vi "Lab Panel V5.27.vi"() -> ()   [LabVIEW 2013] (continued)
                            n3235 = Multiply(x=w5893, y=w5892) -> (x*y=w5891:dbl)
                            n3236 = Multiply(x=w5893, y=w5895) -> (x*y=w5894:dbl)
                          }
                        }
                        n3237 = local read "SIG LAB02-2"() -> (w5885:T2)
                        n3238 = local read "SIG LAB02-1"() -> (w5887:T2)
                        n3239 = Bundle By Name(cluster=w5887, "Tmp Live"=w5867, "Tmp Neut"=w5866) -> (w5886:T2)
                        n3240 = Bundle By Name(cluster=w5885, "Tmp Live"=w5863, "Tmp Neut"=w5862) -> (w5884:T2)
                        n3241 = local write "SIG LAB02-1"(w5886) -> ()
                        n3242 = local write "SIG LAB02-2"(w5884) -> ()
                      }
                      frame #3 {
                        n3243 = case shown="False" w5917 {
                          tunnel: [w5948 w5949] -> w5933
                          tunnel: w5916 -> [_ w5949]
                          frame False {
                            n3244 = local read "CAL LAB03"() -> (w5948:T14)
                          }
                          frame True {
                          }
                        }
                        n3245 = local read "TEMP LA03"() -> (w5923:T9)
                        n3246 = local read "LAB03 TEMP"() -> (w5924:T12)
                        n3247 = call "sub vi - temperature delay v4.vi"("2-run"=w5905, "1-run"=w5906, "temp values IN"=w5923, "temp signals"=w5924) -> ("T2-N"=w5918:dbl, "T2-L"=w5919:dbl, "T1-N"=w5920:dbl, "T1-L"=w5921:dbl, "temp values OUT"=w5922:T44)  [unwired: 3 in]
                        n3248 = Unbundle By Name(w5933) -> ("1 (TL) cal"=w5928:dbl, "1 (TN) cal"=w5927:dbl, "2 (TL) cal"=w5926:dbl, "2 (TN) cal"=w5925:dbl)  [unwired: 6 out]
                        n3249 = local write "TEMP LA03"(w5922) -> ()
                        n3250 = Multiply(x=w5921, y=w5928) -> (x*y=w5914:dbl)
                        n3251 = Multiply(x=w5920, y=w5927) -> (x*y=w5913:dbl)
                        n3252 = Multiply(x=w5919, y=w5926) -> (x*y=w5910:dbl)
                        n3253 = Multiply(x=w5918, y=w5925) -> (x*y=w5909:dbl)
                        n3254 = case shown="True" w5905 {
                          tunnel: w5910 -> [w5935 w5940]
                          tunnel: w5915 -> [_ w5938]
                          tunnel: [w5935 w5939] -> w5908
                          tunnel: w5909 -> [w5934 w5937]
                          tunnel: [w5934 w5936] -> w5907
                          frame False {
                          }
                          frame True {
                            n3255 = Multiply(x=w5938, y=w5937) -> (x*y=w5936:dbl)
                            n3256 = Multiply(x=w5938, y=w5940) -> (x*y=w5939:dbl)
                          }
                        }
                        n3257 = case shown="True" w5906 {
                          tunnel: w5914 -> [w5942 w5947]
                          tunnel: w5915 -> [_ w5945]
                          tunnel: [w5942 w5946] -> w5912
                          tunnel: w5913 -> [w5941 w5944]
                          tunnel: [w5941 w5943] -> w5911
                          frame False {
                          }
                          frame True {
                            n3258 = Multiply(x=w5945, y=w5944) -> (x*y=w5943:dbl)
                            n3259 = Multiply(x=w5945, y=w5947) -> (x*y=w5946:dbl)
                          }
                        }
                        n3260 = local read "SIG LAB03-2"() -> (w5930:T2)
                        n3261 = local read "SIG LAB03-1"() -> (w5932:T2)
                        n3262 = Bundle By Name(cluster=w5932, "Tmp Live"=w5912, "Tmp Neut"=w5911) -> (w5931:T2)
                        n3263 = Bundle By Name(cluster=w5930, "Tmp Live"=w5908, "Tmp Neut"=w5907) -> (w5929:T2)
                        n3264 = local write "SIG LAB03-1"(w5931) -> ()
                        n3265 = local write "SIG LAB03-2"(w5929) -> ()
                      }
                      frame #4 {
                        n3266 = case shown="False" w5962 {
                          tunnel: [w5993 w5994] -> w5978
                          tunnel: w5961 -> [_ w5994]
                          frame False {
                            n3267 = local read "CAL LAB04"() -> (w5993:T14)
                          }
                          frame True {
                          }
                        }
                        n3268 = local read "LAB04 TEMP"() -> (w5968:T12)
                        n3269 = local read "TEMP LA04"() -> (w5969:T9)
                        n3270 = call "sub vi - temperature delay v4.vi"("2-run"=w5950, "1-run"=w5951, "temp values IN"=w5969, "temp signals"=w5968) -> ("T2-N"=w5963:dbl, "T2-L"=w5964:dbl, "T1-N"=w5965:dbl, "T1-L"=w5966:dbl, "temp values OUT"=w5967:T44)  [unwired: 3 in]
                        n3271 = Unbundle By Name(w5978) -> ("1 (TL) cal"=w5973:dbl, "1 (TN) cal"=w5972:dbl, "2 (TL) cal"=w5971:dbl, "2 (TN) cal"=w5970:dbl)  [unwired: 6 out]
                        n3272 = local write "TEMP LA04"(w5967) -> ()
                        n3273 = Multiply(x=w5966, y=w5973) -> (x*y=w5959:dbl)
                        n3274 = Multiply(x=w5965, y=w5972) -> (x*y=w5958:dbl)
                        n3275 = Multiply(x=w5964, y=w5971) -> (x*y=w5955:dbl)
                        n3276 = Multiply(x=w5963, y=w5970) -> (x*y=w5954:dbl)
                        n3277 = case shown="True" w5950 {
                          tunnel: w5955 -> [w5980 w5985]
                          tunnel: w5960 -> [_ w5983]
                          tunnel: [w5980 w5984] -> w5953
                          tunnel: w5954 -> [w5979 w5982]
                          tunnel: [w5979 w5981] -> w5952
                          frame False {
                          }
                          frame True {
                            n3278 = Multiply(x=w5983, y=w5982) -> (x*y=w5981:dbl)
                            n3279 = Multiply(x=w5983, y=w5985) -> (x*y=w5984:dbl)
                          }
                        }
                        n3280 = case shown="True" w5951 {
                          tunnel: w5959 -> [w5987 w5992]
                          tunnel: w5960 -> [_ w5990]
                          tunnel: [w5987 w5991] -> w5957
                          tunnel: w5958 -> [w5986 w5989]
                          tunnel: [w5986 w5988] -> w5956
                          frame False {
                          }
                          frame True {
                            n3281 = Multiply(x=w5990, y=w5989) -> (x*y=w5988:dbl)
                            n3282 = Multiply(x=w5990, y=w5992) -> (x*y=w5991:dbl)
                          }
                        }
                        n3283 = local read "SIG LAB04-2"() -> (w5975:T2)
                        n3284 = local read "SIG LAB04-1"() -> (w5977:T2)
                        n3285 = Bundle By Name(cluster=w5977, "Tmp Live"=w5957, "Tmp Neut"=w5956) -> (w5976:T2)
                        n3286 = Bundle By Name(cluster=w5975, "Tmp Live"=w5953, "Tmp Neut"=w5952) -> (w5974:T2)
                        n3287 = local write "SIG LAB04-1"(w5976) -> ()
                        n3288 = local write "SIG LAB04-2"(w5974) -> ()
                      }
                      frame #5 {
                        n3289 = case shown="False" w6007 {
                          tunnel: [w6038 w6039] -> w6023
                          tunnel: w6006 -> [_ w6039]
                          frame False {
                            n3290 = local read "CAL LAB05"() -> (w6038:T14)
                          }
                          frame True {
                          }
                        }
                        n3291 = local read "LAB05 TEMP"() -> (w6013:T12)
                        n3292 = local read "TEMP LA05"() -> (w6014:T9)
                        n3293 = call "sub vi - temperature delay v4.vi"("2-run"=w5995, "1-run"=w5996, "temp values IN"=w6014, "temp signals"=w6013) -> ("T2-N"=w6009:dbl, "T2-L"=w6010:dbl, "T1-N"=w6011:dbl, "T1-L"=w6012:dbl, "temp values OUT"=w6008:T44)  [unwired: 3 in]
                        n3294 = local write "TEMP LA05"(w6008) -> ()
                        n3295 = Unbundle By Name(w6023) -> ("1 (TL) cal"=w6015:dbl, "1 (TN) cal"=w6018:dbl, "2 (TL) cal"=w6017:dbl, "2 (TN) cal"=w6016:dbl)  [unwired: 6 out]
                        n3296 = Multiply(x=w6012, y=w6015) -> (x*y=w6004:dbl)
                        n3297 = Multiply(x=w6011, y=w6018) -> (x*y=w6003:dbl)
                        n3298 = Multiply(x=w6010, y=w6017) -> (x*y=w6000:dbl)
                        n3299 = Multiply(x=w6009, y=w6016) -> (x*y=w5999:dbl)
                        n3300 = case shown="True" w5995 {
                          tunnel: w6000 -> [w6025 w6030]
                          tunnel: w6005 -> [_ w6028]
                          tunnel: [w6025 w6029] -> w5998
                          tunnel: w5999 -> [w6024 w6027]
                          tunnel: [w6024 w6026] -> w5997
                          frame False {
                          }
                          frame True {
                            n3301 = Multiply(x=w6028, y=w6027) -> (x*y=w6026:dbl)
                            n3302 = Multiply(x=w6028, y=w6030) -> (x*y=w6029:dbl)
                          }
                        }
                        n3303 = case shown="True" w5996 {
                          tunnel: w6004 -> [w6032 w6037]
                          tunnel: w6005 -> [_ w6035]
                          tunnel: [w6032 w6036] -> w6002
                          tunnel: w6003 -> [w6031 w6034]
                          tunnel: [w6031 w6033] -> w6001
                          frame False {
                          }
                          frame True {
                            n3304 = Multiply(x=w6035, y=w6034) -> (x*y=w6033:dbl)
                            n3305 = Multiply(x=w6035, y=w6037) -> (x*y=w6036:dbl)
                          }
                        }
                        n3306 = local read "SIG LAB05-1"() -> (w6022:T2)
                        n3307 = Bundle By Name(cluster=w6022, "Tmp Live"=w6002, "Tmp Neut"=w6001) -> (w6021:T2)
                        n3308 = local read "SIG LAB05-2"() -> (w6020:T2)
                        n3309 = Bundle By Name(cluster=w6020, "Tmp Live"=w5998, "Tmp Neut"=w5997) -> (w6019:T2)
                        n3310 = local write "SIG LAB05-1"(w6021) -> ()
                        n3311 = local write "SIG LAB05-2"(w6019) -> ()
                      }
                      frame #6 {
                        w6140 = 150.0
                        # "check for thermocouple error, output >150 deg??"
                        n3312 = local read "SIG LAB01-2"() -> (w6149:T2)
                        n3313 = local read "SIG LAB04-1"() -> (w6143:T2)
                        n3314 = local read "SIG LAB04-2"() -> (w6144:T2)
                        n3315 = local read "SIG LAB01-1"() -> (w6150:T2)
                        n3316 = Unbundle(w6144) -> ("Tmp Live"=w6054:dbl, "Tmp Neut"=w6053:dbl)  [unwired: 3 out]
                        n3317 = Unbundle(w6149) -> ("Tmp Live"=w6075:dbl, "Tmp Neut"=w6073:dbl)  [unwired: 3 out]
                        n3318 = Unbundle(w6143) -> ("Tmp Live"=w6055:dbl, "Tmp Neut"=w6048:dbl)  [unwired: 3 out]
                        n3319 = Unbundle(w6150) -> ("Tmp Live"=w6078:dbl, "Tmp Neut"=w6076:dbl)  [unwired: 3 out]
                        n3320 = Absolute Value(x=w6055) -> (abs(x)=w6049:dbl)
                        n3321 = Absolute Value(x=w6048) -> (abs(x)=w6050:dbl)
                        n3322 = Absolute Value(x=w6054) -> (abs(x)=w6052:dbl)
                        n3323 = Absolute Value(x=w6053) -> (abs(x)=w6051:dbl)
                        n3324 = Absolute Value(x=w6075) -> (abs(x)=w6074:dbl)
                        n3325 = Absolute Value(x=w6073) -> (abs(x)=w6072:dbl)
                        n3326 = Absolute Value(x=w6076) -> (abs(x)=w6077:dbl)
                        n3327 = Absolute Value(x=w6078) -> (abs(x)=w6079:dbl)
                        n3328 = Greater?(x=w6051, y=w6140) -> (0:w6116:bool)
                        "LA04-2 (TN)" <- w6116
                        n3329 = Greater?(x=w6072, y=w6140) -> (0:w6128:bool)
                        "LA01-2 (TN)" <- w6128
                        n3330 = Greater?(x=w6052, y=w6140) -> (0:w6117:bool)
                        "LA04-2 (TL)" <- w6117
                        n3331 = Greater?(x=w6074, y=w6140) -> (0:w6129:bool)
                        "LA01-2 (TL)" <- w6129
                        n3332 = Greater?(x=w6050, y=w6140) -> (0:w6118:bool)
                        "LA04-1 (TN)" <- w6118
                        n3333 = Greater?(x=w6077, y=w6140) -> (0:w6139:bool)
                        "LA01-1 (TN)" <- w6139
                        n3334 = Greater?(x=w6049, y=w6140) -> (0:w6119:bool)
                        "LA04-1 (TL)" <- w6119
                        n3335 = Greater?(x=w6079, y=w6140) -> (0:w6138:bool)
                        "LA01-1 (TL)" <- w6138
                        n3336 = Or(x=w6139, y=w6138) -> (x .or. y?=w6137:bool)
                        n3337 = Or(x=w6116, y=w6117) -> (x .or. y?=w6127:bool)
                        n3338 = Or(x=w6129, y=w6128) -> (x .or. y?=w6133:bool)
                        n3339 = Or(x=w6118, y=w6119) -> (x .or. y?=w6123:bool)
                        n3340 = Select(t=u32 16711680, s=w6137, f=u32 13816530) -> (s? t:f=w6134:u32)
                        n3341 = Select(t=u32 16711680, s=w6127, f=u32 13816530) -> (s? t:f=w6124:u32)
                        n3342 = Select(t=u32 16711680, s=w6133, f=u32 13816530) -> (s? t:f=w6130:u32)
                        n3343 = Select(t=u32 16711680, s=w6123, f=u32 13816530) -> (s? t:f=w6120:u32)
                        n3344 = property on="SIG LAB01-1" class="Clust (strict)"("Color"=w6134) -> ()  [unwired: 2 in, 2 out]
                        n3345 = property on="SIG LAB01-2" class="Clust (strict)"("Color"=w6130) -> ()  [unwired: 2 in, 2 out]
                        n3346 = property on="SIG LAB04-2" class="Clust (strict)"("Color"=w6124) -> ()  [unwired: 2 in, 2 out]
                        n3347 = property on="SIG LAB04-1" class="Clust (strict)"("Color"=w6120) -> ()  [unwired: 2 in, 2 out]
                        n3348 = local read "SIG LAB02-1"() -> (w6147:T2)
                        n3349 = local read "SIG LAB02-2"() -> (w6148:T2)
                        n3350 = local read "SIG LAB05-2"() -> (w6141:T2)
                        n3351 = local read "SIG LAB05-1"() -> (w6142:T2)
                        n3352 = Unbundle(w6148) -> ("Tmp Live"=w6067:dbl, "Tmp Neut"=w6065:dbl)  [unwired: 3 out]
                        n3353 = Unbundle(w6147) -> ("Tmp Live"=w6071:dbl, "Tmp Neut"=w6070:dbl)  [unwired: 3 out]
                        n3354 = Unbundle(w6141) -> ("Tmp Live"=w6043:dbl, "Tmp Neut"=w6041:dbl)  [unwired: 3 out]
                        n3355 = Unbundle(w6142) -> ("Tmp Live"=w6047:dbl, "Tmp Neut"=w6045:dbl)  [unwired: 3 out]
                        n3356 = Absolute Value(x=w6067) -> (abs(x)=w6066:dbl)
                        n3357 = Absolute Value(x=w6065) -> (abs(x)=w6064:dbl)
                        n3358 = Absolute Value(x=w6070) -> (abs(x)=w6068:dbl)
                        n3359 = Absolute Value(x=w6071) -> (abs(x)=w6069:dbl)
                        n3360 = Absolute Value(x=w6043) -> (abs(x)=w6042:dbl)
                        n3361 = Absolute Value(x=w6041) -> (abs(x)=w6040:dbl)
                        n3362 = Absolute Value(x=w6047) -> (abs(x)=w6046:dbl)
                        n3363 = Absolute Value(x=w6045) -> (abs(x)=w6044:dbl)
                        n3364 = Greater?(x=w6064, y=w6140) -> (0:w6092:bool)
                        "LA02-2 (TN)" <- w6092
                        n3365 = Greater?(x=w6066, y=w6140) -> (0:w6093:bool)
                        "LA02-2 (TL)" <- w6093
                        n3366 = Greater?(x=w6068, y=w6140) -> (0:w6095:bool)
                        "LA02-1 (TN)" <- w6095
                        n3367 = Greater?(x=w6069, y=w6140) -> (0:w6094:bool)
                        "LA02-1 (TL)" <- w6094
                        n3368 = Greater?(x=w6040, y=w6140) -> (0:w6104:bool)
                        "LA05-2 (TN)" <- w6104
                        n3369 = Greater?(x=w6042, y=w6140) -> (0:w6105:bool)
                        "LA05-2 (TL)" <- w6105
                        n3370 = Greater?(x=w6044, y=w6140) -> (0:w6106:bool)
                        "LA05-1 (TN)" <- w6106
                        n3371 = Greater?(x=w6046, y=w6140) -> (0:w6107:bool)
                        "LA05-1 (TL)" <- w6107
                        n3372 = Or(x=w6095, y=w6094) -> (x .or. y?=w6103:bool)
                        n3373 = Or(x=w6093, y=w6092) -> (x .or. y?=w6099:bool)
                        n3374 = Or(x=w6107, y=w6106) -> (x .or. y?=w6115:bool)
                        n3375 = Or(x=w6105, y=w6104) -> (x .or. y?=w6111:bool)
                        n3376 = Select(t=u32 16711680, s=w6103, f=u32 13816530) -> (s? t:f=w6100:u32)
                        n3377 = Select(t=u32 16711680, s=w6099, f=u32 13816530) -> (s? t:f=w6096:u32)
                        n3378 = Select(t=u32 16711680, s=w6115, f=u32 13816530) -> (s? t:f=w6112:u32)
                        n3379 = Select(t=u32 16711680, s=w6111, f=u32 13816530) -> (s? t:f=w6108:u32)
                        n3380 = local read "SIG LAB03-1"() -> (w6145:T2)
                        n3381 = property on="SIG LAB02-1" class="Clust (strict)"("Color"=w6100) -> ()  [unwired: 2 in, 2 out]
                        n3382 = property on="SIG LAB02-2" class="Clust (strict)"("Color"=w6096) -> ()  [unwired: 2 in, 2 out]
                        n3383 = local read "SIG LAB03-2"() -> (w6146:T2)
                        n3384 = property on="SIG LAB05-1" class="Clust (strict)"("Color"=w6112) -> ()  [unwired: 2 in, 2 out]
                        n3385 = property on="SIG LAB05-2" class="Clust (strict)"("Color"=w6108) -> ()  [unwired: 2 in, 2 out]
                        n3386 = Unbundle(w6146) -> ("Tmp Live"=w6059:dbl, "Tmp Neut"=w6057:dbl)  [unwired: 3 out]
                        n3387 = Unbundle(w6145) -> ("Tmp Live"=w6063:dbl, "Tmp Neut"=w6061:dbl)  [unwired: 3 out]
                        n3388 = Absolute Value(x=w6059) -> (abs(x)=w6058:dbl)
                        n3389 = Absolute Value(x=w6057) -> (abs(x)=w6056:dbl)
                        n3390 = Absolute Value(x=w6063) -> (abs(x)=w6062:dbl)
                        n3391 = Absolute Value(x=w6061) -> (abs(x)=w6060:dbl)
                        n3392 = Greater?(x=w6056, y=w6140) -> (0:w6080:bool)
                        "LA03-2 (TN)" <- w6080
                        n3393 = Greater?(x=w6058, y=w6140) -> (0:w6081:bool)
                        "LA03-2 (TL)" <- w6081
                        n3394 = Greater?(x=w6060, y=w6140) -> (0:w6083:bool)
                        "LA03-1 (TN)" <- w6083
                        n3395 = Greater?(x=w6062, y=w6140) -> (0:w6082:bool)
                        "LA03-1 (TL)" <- w6082
                        n3396 = Or(x=w6083, y=w6082) -> (x .or. y?=w6091:bool)
                        n3397 = Or(x=w6081, y=w6080) -> (x .or. y?=w6087:bool)
                        n3398 = Select(t=u32 16711680, s=w6091, f=u32 13816530) -> (s? t:f=w6088:u32)
                        n3399 = Select(t=u32 16711680, s=w6087, f=u32 13816530) -> (s? t:f=w6084:u32)
                        n3400 = property on="SIG LAB03-1" class="Clust (strict)"("Color"=w6088) -> ()  [unwired: 2 in, 2 out]
                        n3401 = property on="SIG LAB03-2" class="Clust (strict)"("Color"=w6084) -> ()  [unwired: 2 in, 2 out]
                      }
                    }
                  }
                }
              }
            }
          }
          frame #22 {
            # "SAVE ON AMPS VALUES FOR REPORT FILE"
            # "write data to display panel"
            n3402 = global write "Global display 1.vi" "TEST 5-2"(w6186) -> ()
            n3403 = global write "Global display 1.vi" "TEST 4-2"(w6188) -> ()
            n3404 = global write "Global display 1.vi" "TEST 1-2"(w6194) -> ()
            n3405 = global write "Global display 1.vi" "TEST 3-1"(w6191) -> ()
            n3406 = global write "Global display 1.vi" "TEST 5-1"(w6187) -> ()
            n3407 = global write "Global display 1.vi" "TEST 1-1"(w6195) -> ()
            n3408 = global write "Global display 1.vi" "TEST 3-2"(w6190) -> ()
            n3409 = global write "Global display 1.vi" "TEST 4-1"(w6189) -> ()
            n3410 = global write "Global display 1.vi" "TEST 2-2"(w6192) -> ()
            n3411 = global write "Global display 1.vi" "TEST 2-1"(w6193) -> ()
            n3412 = global read "Global display 3.vi" "log 1-1"() -> (→"LOG LAB01-1":string)
            n3413 = global read "Global display 3.vi" "log 3-1"() -> (→"LOG LAB03-1":string)
            n3414 = global read "Global display 3.vi" "log 1-2"() -> (→"LOG LAB01-2":string)
            n3415 = property on="Tab Control 2" class="TabCtl (strict)"() -> ("Pages"=w6185:refnum<vi>[])  [unwired: 2 in, 2 out]
            n3416 = global read "Global display 3.vi" "log 2-1"() -> (→"LOG LAB02-1":string)
            n3417 = global read "Global display 3.vi" "log 2-2"() -> (→"LOG LAB02-2":string)
            n3418 = global read "Global display 3.vi" "log 4-2"() -> (→"LOG LAB04-2":string)
            n3419 = global read "Global display 3.vi" "log 5-2"() -> (→"LOG LAB05-2":string)
            n3420 = global read "Global display 3.vi" "log 5-1"() -> (→"LOG LAB05-1":string)
            n3421 = global read "Global display 3.vi" "log 4-1"() -> (→"LOG LAB04-1":string)
            n3422 = global read "Global display 3.vi" "log 3-2"() -> (→"LOG LAB03-2":string)
            n3423 = Index Array(array=w6185, index=8) -> (element=w6183:refnum<vi>)
            n3424 = property class="Page"(reference=w6183) -> ("PageVis"=w6182:bool)  [unwired: 1 in, 2 out]
            n3425 = global write "Global display 3.vi" "admin"(w6182) -> ()
            n3426 = local read "O/I  LAB05-2"() -> (w6236:bool)
            n3427 = local read "O/I  LAB05-1"() -> (w6237:bool)
            n3428 = local read "O/I  LAB03-2"() -> (w6240:bool)
            n3429 = local read "O/I  LAB04-2"() -> (w6238:bool)
            n3430 = local read "O/I  LAB04-1"() -> (w6239:bool)
            n3431 = local read "O/I  LAB03-1"() -> (w6241:bool)
            n3432 = local read "O/I  LAB01-2"() -> (w6244:bool)
            n3433 = local read "O/I  LAB01-1"() -> (w6245:bool)
            n3434 = local read "O/I  LAB02-1"() -> (w6243:bool)
            n3435 = local read "O/I  LAB02-2"() -> (w6242:bool)
            n3436 = global write "Global display 1.vi" "5-2 O/F"(w6236) -> ()
            n3437 = global write "Global display 1.vi" "5-1 O/F"(w6237) -> ()
            n3438 = global write "Global display 1.vi" "4-1 O/F"(w6239) -> ()
            n3439 = global write "Global display 1.vi" "4-2 O/F"(w6238) -> ()
            n3440 = global write "Global display 1.vi" "3-2 O/F"(w6240) -> ()
            n3441 = global write "Global display 1.vi" "3-1 O/F"(w6241) -> ()
            n3442 = global write "Global display 1.vi" "2-2 O/F"(w6242) -> ()
            n3443 = global write "Global display 1.vi" "2-1 O/F"(w6243) -> ()
            n3444 = global write "Global display 1.vi" "1-2 O/F"(w6244) -> ()
            n3445 = global write "Global display 1.vi" "1-1 O/F"(w6245) -> ()
            n3446 = local read "TEMP START LAB02-2"() -> (w6168:cluster{"TL":dbl, "TN":dbl})
            n3447 = local read "run lab05-2"() -> (w6226:bool)
            n3448 = local read "TEMP START LAB01-2"() -> (w6170:cluster{"TL":dbl, "TN":dbl})
            n3449 = local read "TEMP START LAB02-1"() -> (w6169:cluster{"TL":dbl, "TN":dbl})
            n3450 = local read "TEMP START LAB04-1"() -> (w6165:cluster{"TL":dbl, "TN":dbl})
            n3451 = local read "TEMP START LAB04-2"() -> (w6164:cluster{"TL":dbl, "TN":dbl})
            n3452 = local read "run lab04-1"() -> (w6229:bool)
            n3453 = local read "run lab04-2"() -> (w6228:bool)
            n3454 = local read "run lab05-1"() -> (w6227:bool)
            n3455 = local read "TEMP START LAB01-1"() -> (w6171:cluster{"TL":dbl, "TN":dbl})
            n3456 = local read "TEMP START LAB05-2"() -> (w6162:cluster{"TL":dbl, "TN":dbl})
            n3457 = local read "TEMP START LAB05-1"() -> (w6163:cluster{"TL":dbl, "TN":dbl})
            n3458 = local read "run lab03-2"() -> (w6230:bool)
            n3459 = local read "TEMP START LAB03-2"() -> (w6166:cluster{"TL":dbl, "TN":dbl})
            n3460 = local read "TEMP START LAB03-1"() -> (w6167:cluster{"TL":dbl, "TN":dbl})
            n3461 = local read "run lab02-1"() -> (w6233:bool)
            n3462 = local read "run lab03-1"() -> (w6231:bool)
            n3463 = local read "run lab01-2"() -> (w6234:bool)
            n3464 = local read "run lab02-2"() -> (w6232:bool)
            n3465 = local read "run lab01-1"() -> (w6235:bool)
            n3466 = global write "Global display 1.vi" "5-2 R/S"(w6226) -> ()
            n3467 = global write "Global display 1.vi" "5-1 R/S"(w6227) -> ()
            n3468 = global write "Global display 1.vi" "4-2 R/S"(w6228) -> ()
            n3469 = global write "Global display 1.vi" "4-1 R/S"(w6229) -> ()
            n3470 = global write "Global display 1.vi" "3-2 R/S"(w6230) -> ()
            n3471 = global write "Global display 1.vi" "1-2 R/S"(w6234) -> ()
            n3472 = global write "Global display 1.vi" "2-1 R/S"(w6233) -> ()
            n3473 = global write "Global display 1.vi" "3-1 R/S"(w6231) -> ()
            n3474 = global write "Global display 1.vi" "2-2 R/S"(w6232) -> ()
            n3475 = global write "Global display 1.vi" "1-1 R/S"(w6235) -> ()
            n3476 = global write "Global display 3.vi" "TEMP ST 05-2"(w6162) -> ()
            n3477 = global write "Global display 3.vi" "TEMP ST 05-1"(w6163) -> ()
            n3478 = global write "Global display 3.vi" "TEMP ST 03-2"(w6166) -> ()
            n3479 = global write "Global display 3.vi" "TEMP ST 04-2"(w6164) -> ()
            n3480 = global write "Global display 3.vi" "TEMP ST 01-1"(w6171) -> ()
            n3481 = global write "Global display 3.vi" "TEMP ST 01-2"(w6170) -> ()
            n3482 = global write "Global display 3.vi" "TEMP ST 04-1"(w6165) -> ()
            n3483 = global write "Global display 3.vi" "TEMP ST 02-1"(w6169) -> ()
            n3484 = global write "Global display 3.vi" "TEMP ST 02-2"(w6168) -> ()
            n3485 = global write "Global display 3.vi" "TEMP ST 03-1"(w6167) -> ()
            n3486 = local read "DISP LAB04-2"() -> (w6218:T4)
            n3487 = local read "DISP LAB05-1"() -> (w6217:T4)
            n3488 = local read "DISP LAB04-1"() -> (w6219:T4)
            n3489 = local read "DISP LAB05-2"() -> (w6216:T4)
            n3490 = local read "DISP LAB03-2"() -> (w6220:T4)
            n3491 = local read "DISP LAB03-1"() -> (w6221:T4)
            n3492 = local read "DISP LAB01-2"() -> (w6224:T4)
            n3493 = local read "DISP LAB02-1"() -> (w6223:T4)
            n3494 = local read "DISP LAB02-2"() -> (w6222:T4)
            n3495 = local read "DISP LAB01-1"() -> (w6225:T4)
            n3496 = local read "TEMP RISE LAB05-1"() -> (w6153:cluster{"TL":dbl, "TN":dbl})
            n3497 = local read "TEMP RISE LAB05-2"() -> (w6152:cluster{"TL":dbl, "TN":dbl})
            n3498 = local read "TEMP RISE LAB04-2"() -> (w6154:cluster{"TL":dbl, "TN":dbl})
            n3499 = local read "TEMP RISE LAB04-1"() -> (w6155:cluster{"TL":dbl, "TN":dbl})
            n3500 = local read "TEMP RISE LAB03-2"() -> (w6156:cluster{"TL":dbl, "TN":dbl})
            n3501 = local read "TEMP RISE LAB03-1"() -> (w6157:cluster{"TL":dbl, "TN":dbl})
            n3502 = local read "TEMP RISE LAB01-2"() -> (w6160:cluster{"TL":dbl, "TN":dbl})
            n3503 = local read "TEMP RISE LAB02-2"() -> (w6158:cluster{"TL":dbl, "TN":dbl})
            n3504 = local read "TEMP RISE LAB01-1"() -> (w6161:cluster{"TL":dbl, "TN":dbl})
            n3505 = local read "TEMP RISE LAB02-1"() -> (w6159:cluster{"TL":dbl, "TN":dbl})
            n3506 = global write "Global display 2.vi" "DISP LAB05-1"(w6217) -> ()
            n3507 = global write "Global display 2.vi" "DISP LAB05-2"(w6216) -> ()
            n3508 = global write "Global display 2.vi" "DISP LAB04-2"(w6218) -> ()
            n3509 = global write "Global display 2.vi" "DISP LAB04-1"(w6219) -> ()
            n3510 = global write "Global display 2.vi" "DISP LAB02-1"(w6223) -> ()
            n3511 = global write "Global display 2.vi" "DISP LAB02-2"(w6222) -> ()
            n3512 = global write "Global display 2.vi" "DISP LAB03-2"(w6220) -> ()
            n3513 = global write "Global display 2.vi" "DISP LAB01-2"(w6224) -> ()
            n3514 = global write "Global display 2.vi" "DISP LAB01-1"(w6225) -> ()
            n3515 = global write "Global display 2.vi" "DISP LAB03-1"(w6221) -> ()
            n3516 = global write "Global display 3.vi" "TEMP RS 05-2"(w6152) -> ()
            n3517 = global write "Global display 3.vi" "TEMP RS 05-1"(w6153) -> ()
            n3518 = global write "Global display 3.vi" "TEMP RS 03-2"(w6156) -> ()
            n3519 = global write "Global display 3.vi" "TEMP RS 02-1"(w6159) -> ()
            n3520 = global write "Global display 3.vi" "TEMP RS 02-2"(w6158) -> ()
            n3521 = global write "Global display 3.vi" "TEMP RS 04-2"(w6154) -> ()
            n3522 = global write "Global display 3.vi" "TEMP RS 01-2"(w6160) -> ()
            n3523 = global write "Global display 3.vi" "TEMP RS 03-1"(w6157) -> ()
            n3524 = global write "Global display 3.vi" "TEMP RS 04-1"(w6155) -> ()
            n3525 = global write "Global display 3.vi" "TEMP RS 01-1"(w6161) -> ()
            n3526 = local read "SET LAB05-2"() -> (w6206:T5)
            n3527 = local read "SET LAB05-1"() -> (w6207:T5)
            n3528 = local read "SET LAB04-1"() -> (w6209:T5)
            n3529 = local read "SET LAB04-2"() -> (w6208:T5)
            n3530 = local read "SET LAB01-1"() -> (w6215:T5)
            n3531 = local read "SET LAB03-1"() -> (w6211:T5)
            n3532 = local read "SET LAB03-2"() -> (w6210:T5)
            n3533 = local read "SET LAB02-2"() -> (w6212:T5)
            n3534 = local read "SET LAB01-2"() -> (w6214:T5)
            n3535 = local read "SET LAB02-1"() -> (w6213:T5)
            n3536 = global write "Global display 2.vi" "SET LAB05-2"(w6206) -> ()
            n3537 = global write "Global display 2.vi" "SET LAB05-1"(w6207) -> ()
            n3538 = global write "Global display 2.vi" "SET LAB04-1"(w6209) -> ()
            n3539 = global write "Global display 2.vi" "SET LAB01-1"(w6215) -> ()
            n3540 = global write "Global display 2.vi" "SET LAB04-2"(w6208) -> ()
            n3541 = global write "Global display 2.vi" "SET LAB03-2"(w6210) -> ()
            n3542 = global write "Global display 2.vi" "SET LAB02-2"(w6212) -> ()
            n3543 = global write "Global display 2.vi" "SET LAB03-1"(w6211) -> ()
            n3544 = global write "Global display 2.vi" "SET LAB01-2"(w6214) -> ()
            n3545 = global write "Global display 2.vi" "SET LAB02-1"(w6213) -> ()
            n3546 = local read "RESULT LAB01-1"() -> (w6205:bool)
            n3547 = local read "RESULT LAB03-2"() -> (w6200:bool)
            n3548 = local read "RESULT LAB04-1"() -> (w6199:bool)
            n3549 = local read "RESULT LAB04-2"() -> (w6198:bool)
            n3550 = local read "RESULT LAB02-2"() -> (w6202:bool)
            n3551 = local read "RESULT LAB01-2"() -> (w6204:bool)
            n3552 = local read "RESULT LAB02-1"() -> (w6203:bool)
            n3553 = local read "RESULT LAB03-1"() -> (w6201:bool)
            n3554 = local read "RESULT LAB05-1"() -> (w6197:bool)
            n3555 = local read "RESULT LAB05-2"() -> (w6196:bool)
            n3556 = global write "Global display 2.vi" "RESULT LAB05-1"(w6197) -> ()
            n3557 = global write "Global display 2.vi" "RESULT LAB01-2"(w6204) -> ()
            n3558 = global write "Global display 2.vi" "RESULT LAB03-2"(w6200) -> ()
            n3559 = global write "Global display 2.vi" "RESULT LAB04-1"(w6199) -> ()
            n3560 = global write "Global display 2.vi" "RESULT LAB04-2"(w6198) -> ()
            n3561 = global write "Global display 2.vi" "RESULT LAB05-2"(w6196) -> ()
            n3562 = global write "Global display 2.vi" "RESULT LAB03-1"(w6201) -> ()
            n3563 = global write "Global display 2.vi" "RESULT LAB02-1"(w6203) -> ()
            n3564 = global write "Global display 2.vi" "RESULT LAB02-2"(w6202) -> ()
            n3565 = global write "Global display 2.vi" "RESULT LAB01-1"(w6205) -> ()
            n3566 = local read "Amps Fail level"() -> (w6151:dbl)
            n3567 = stacked-sequence {
              tunnel: w6151 -> [w6247 w6252 w6257 w6262 w6267 w6272 w6277 w6282 w6287 w6292]
              frame #0 {
                n3568 = local read "SIG LAB01-1"() -> (w6249:T2)
                n3569 = Unbundle(w6249) -> ("AMPS"=w6248:dbl)  [unwired: 4 out]
                n3570 = Greater?(x=w6248, y=w6247) -> (0:w6246:bool)
                n3571 = case shown="True" w6246 {
                  frame False {
                  }
                  frame True {
                    n3572 = local read "ON L01-1"() -> (w6250:cluster{"amps":dbl, "volts":dbl, "pf":dbl})
                    n3573 = global write "Global display 2.vi" "ON L01-1"(w6250) -> ()
                  }
                }
              }
              frame #1 {
                n3574 = local read "SIG LAB01-2"() -> (w6254:T2)
                n3575 = Unbundle(w6254) -> ("AMPS"=w6253:dbl)  [unwired: 4 out]
                n3576 = Greater?(x=w6253, y=w6252) -> (0:w6251:bool)
                n3577 = case shown="True" w6251 {
                  frame False {
                  }
                  frame True {
                    n3578 = local read "ON L01-2"() -> (w6255:cluster{"amps":dbl, "volts":dbl, "pf":dbl})
                    n3579 = global write "Global display 2.vi" "ON L01-2"(w6255) -> ()
                  }
                }
              }
              frame #2 {
                n3580 = local read "SIG LAB02-1"() -> (w6259:T2)
                n3581 = Unbundle(w6259) -> ("AMPS"=w6258:dbl)  [unwired: 4 out]
                n3582 = Greater?(x=w6258, y=w6257) -> (0:w6256:bool)
                n3583 = case shown="True" w6256 {
                  frame False {
                  }
                  frame True {
                    n3584 = local read "ON L02-1"() -> (w6260:cluster{"amps":dbl, "volts":dbl, "pf":dbl})
                    n3585 = global write "Global display 2.vi" "ON L02-1"(w6260) -> ()
                  }
                }
              }
              frame #3 {
                n3586 = local read "SIG LAB02-2"() -> (w6264:T2)
                n3587 = Unbundle(w6264) -> ("AMPS"=w6263:dbl)  [unwired: 4 out]
                n3588 = Greater?(x=w6263, y=w6262) -> (0:w6261:bool)
                n3589 = case shown="True" w6261 {
                  frame False {
                  }
                  frame True {
                    n3590 = local read "ON L02-2"() -> (w6265:cluster{"amps":dbl, "volts":dbl, "pf":dbl})
                    n3591 = global write "Global display 2.vi" "ON L02-2"(w6265) -> ()
                  }
                }
              }
              frame #4 {
                n3592 = local read "SIG LAB03-1"() -> (w6269:T2)
                n3593 = Unbundle(w6269) -> ("AMPS"=w6268:dbl)  [unwired: 4 out]
                n3594 = Greater?(x=w6268, y=w6267) -> (0:w6266:bool)
                n3595 = case shown="True" w6266 {
                  frame False {
                  }
                  frame True {
                    n3596 = local read "ON L03-1"() -> (w6270:cluster{"amps":dbl, "volts":dbl, "pf":dbl})
                    n3597 = global write "Global display 2.vi" "ON L03-1"(w6270) -> ()
                  }
                }
              }
              frame #5 {
                n3598 = local read "SIG LAB03-2"() -> (w6274:T2)
                n3599 = Unbundle(w6274) -> ("AMPS"=w6273:dbl)  [unwired: 4 out]
                n3600 = Greater?(x=w6273, y=w6272) -> (0:w6271:bool)
                n3601 = case shown="True" w6271 {
                  frame False {
                  }
                  frame True {
                    n3602 = local read "ON L03-2"() -> (w6275:cluster{"amps":dbl, "volts":dbl, "pf":dbl})
                    n3603 = global write "Global display 2.vi" "ON L03-2"(w6275) -> ()
                  }
                }
              }
              frame #6 {
                n3604 = local read "SIG LAB04-1"() -> (w6279:T2)
                n3605 = Unbundle(w6279) -> ("AMPS"=w6278:dbl)  [unwired: 4 out]
                n3606 = Greater?(x=w6278, y=w6277) -> (0:w6276:bool)
                n3607 = case shown="True" w6276 {
                  frame False {
                  }
                  frame True {
                    n3608 = local read "ON L04-1"() -> (w6280:cluster{"amps":dbl, "volts":dbl, "pf":dbl})
                    n3609 = global write "Global display 2.vi" "ON L04-1"(w6280) -> ()
                  }
                }
              }
              frame #7 {
                n3610 = local read "SIG LAB04-2"() -> (w6284:T2)
                n3611 = Unbundle(w6284) -> ("AMPS"=w6283:dbl)  [unwired: 4 out]
                n3612 = Greater?(x=w6283, y=w6282) -> (0:w6281:bool)
                n3613 = case shown="True" w6281 {
                  frame False {
                  }
                  frame True {
                    n3614 = local read "ON L04-2"() -> (w6285:cluster{"amps":dbl, "volts":dbl, "pf":dbl})
                    n3615 = global write "Global display 2.vi" "ON L04-2"(w6285) -> ()
                  }
                }
              }
              frame #8 {
                n3616 = local read "SIG LAB05-1"() -> (w6289:T2)
                n3617 = Unbundle(w6289) -> ("AMPS"=w6288:dbl)  [unwired: 4 out]
                n3618 = Greater?(x=w6288, y=w6287) -> (0:w6286:bool)
                n3619 = case shown="True" w6286 {
                  frame False {
                  }
                  frame True {
                    n3620 = local read "ON L05-1"() -> (w6290:cluster{"amps":dbl, "volts":dbl, "pf":dbl})
                    n3621 = global write "Global display 2.vi" "ON L05-1"(w6290) -> ()
                  }
                }
              }
              frame #9 {
                n3622 = local read "SIG LAB05-2"() -> (w6294:T2)
                n3623 = Unbundle(w6294) -> ("AMPS"=w6293:dbl)  [unwired: 4 out]
                n3624 = Greater?(x=w6293, y=w6292) -> (0:w6291:bool)
                n3625 = case shown="True" w6291 {
                  frame False {
                  }
                  frame True {
                    n3626 = local read "ON L05-2"() -> (w6295:cluster{"amps":dbl, "volts":dbl, "pf":dbl})
                    n3627 = global write "Global display 2.vi" "ON L05-2"(w6295) -> ()
                  }
                }
              }
            }
          }
          frame #23 {
            # "simulate values"
            n3628 = global write "Global display 4.vi" "LAB deg C"("LAB deg C") -> ()
          }
          frame #24 {
            # "end main and display program"
            n3629 = stacked-sequence {
              seq-local: [_ w6302 _] -> [_ _ w6308]
              tunnel: w6298 -> [w6299 _ _]
              tunnel: w6297 -> [_ _ w6306]
              frame #0 {
                n3630 = case shown="True" w6299 {
                  frame False {
                  }
                  frame True {
                    n3631 = One Button Dialog(message="Excessive number of USB \nresets done, re-start program.") -> ()  [unwired: 1 in, 1 out]
                  }
                }
              }
              frame #1 {
                # "check for reset error"
                n3632 = local read "Simulate"() -> (w6301:bool)
                n3633 = case shown="False" w6301 {
                  tunnel: [w6303 FALSE] -> w6302
                  frame False {
                    n3634 = local read "Reset Error"() -> (w6303:bool)
                    n3635 = case shown="True" w6303 {
                      frame False {
                      }
                      frame True {
                        n3636 = One Button Dialog(message="USB ERROR, program will be stopped.\nClose program, close windows, switch panel off\nand re power panel. If error persists seek help.") -> ()  [unwired: 1 in, 1 out]
                      }
                    }
                  }
                  frame True {
                  }
                }
              }
              frame #2 {
                # "end labview session"
                n3637 = case shown="True" w6306 {
                  frame False {
                  }
                  frame True {
                    n3638 = local read "AI Task2"() -> (w6312:dbl)
                    n3639 = local read "AI Task1"() -> (w6311:dbl)
                    n3640 = local read "AI Task0"() -> (w6310:dbl)
                    n3641 = call "sub vi - AI USB4704 (3)  Close Task v1.vi"("TASK USB 0"=w6310, "TASK USB 1"=w6311, "TASK USB 2"=w6312) -> ()  [unwired: 13 in]
                  }
                }
                n3642 = Or(x=w6308, y="stop all") -> (x .or. y?=w6307:bool)
                n3643 = case shown="True" w6307 {
                  frame False {
                  }
                  frame True {
                    n3644 = stacked-sequence {
                      frame #0 {
                        n3645 = global write "Global display 1.vi" "stop disp"(TRUE) -> ()
                      }
                      frame #1 {
                        n3646 = local read "AI Task2"() -> (w6314:dbl)
                        n3647 = local read "AI Task1"() -> (w6315:dbl)
                        n3648 = local read "AI Task0"() -> (w6316:dbl)
                        n3649 = call "sub vi - AI USB4704 (3)  Close Task v1.vi"("TASK USB 0"=w6316, "TASK USB 1"=w6315, "TASK USB 2"=w6314) -> ()  [unwired: 13 in]
                      }
                      frame #2 {
                        n3650 = Quit LabVIEW(quit? (T)=TRUE) -> ()
                      }
                    }
                  }
                }
              }
            }
          }
        }
        n3651 = node-c288() -> ()  [unwired: 1 in, 1 out]
        "loops" <- w350
      }
      n3652 = node-c288(w322) -> ()  [unwired: 1 out]
    }
  }
